vi "H5Sselect_hyperslab.vi"(4 "Count":u64[](array[numeric]), 5 "Block":u64[](array[numeric]), 6 "Start":u64[](array[numeric]), 7 "Stride":u64[](array[numeric]), 8 "error in (no error)":errorcluster, 10 "Operator":T1 items=["H5S_SELECT_NOOP"=-1, "H5S_SELECT_SET"=0, "H5S_SELECT_OR"=1, "H5S_SELECT_AND"=2, "H5S_SELECT_XOR"=3, "H5S_SELECT_NOTB"=4, "H5S_SELECT_NOTA"=5, "H5S_SELECT_APPEND"=6, "H5S_SELECT_PREPEND"=7], 11 "HDF5 Space Ref":T2) -> (0 "error out":errorcluster, 3 "HDF5 Ref out":T2)   [LabVIEW 2017]
doc: "Selects a hyperslab region to add to the current selected region."
uses:
  <vilib>/UPVI/lvhdf5/library.llb/HDF5 Ref.ctl
  <vilib>/UPVI/lvhdf5/dataspace.llb/H5S_seloper_t.ctl
  <vilib>/UPVI/lvhdf5/hdf5.dll
panel:
  # "LVHDF5 Toolkit\nCopyright (c) 2005-2013 by Jason D. Sommerville\nCopyright (c) 2014 by UPVI, LLC.\n\nThis use and distribution of this file is governed by the terms found in \nLICENSE.txt distributed with this toolkit and installed at\n <user.lib>\\_lvhdf5\\LICENSE.txt"
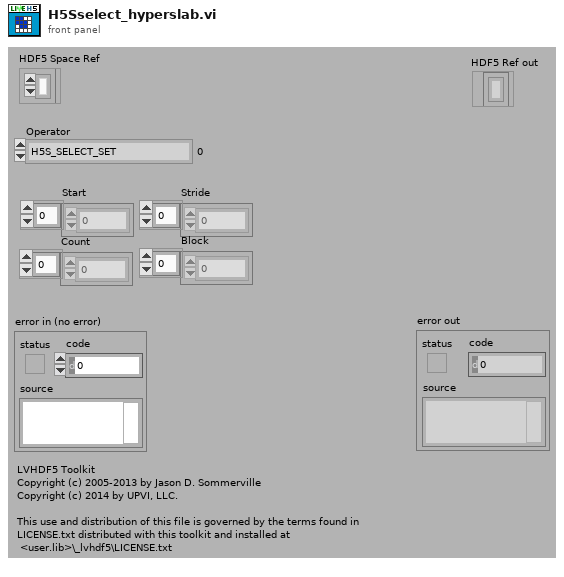
[diagram p1: front panel]
types:
  T1 = typedef "H5S_seloper_t.ctl" = i32
  T2 = typedef "HDF5 Ref.ctl" = refnum<k1>
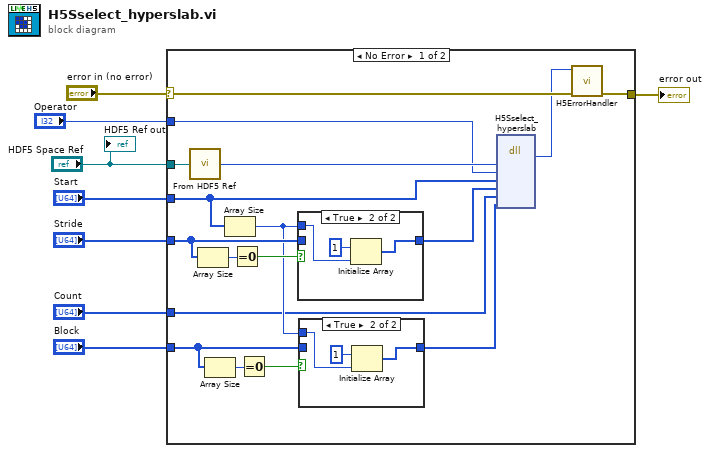
[diagram p0: block diagram]
diagram:
  n1 = case shown="No Error" "error in (no error)" {
    selector: "error in (no error)" -> [w25 w34]
    tunnel: [w24 w34] -> w7
    tunnel: "HDF5 Space Ref" -> [w23 _]
    tunnel: "Operator" -> [w20 _]
    tunnel: "Start" -> [w10 _]
    tunnel: "Stride" -> [w17 _]
    tunnel: "Count" -> [w12 _]
    tunnel: "Block" -> [w15 _]
    frame No Error {
      n2 = call <vilib>:"From HDF5 Ref.vi"("HDF5 Ref"=w23) -> ("I32"=w22:i32)
      n3 = Array Size(array=w17) -> (size(s)=w19:i32)
      n4 = Array Size(array=w15) -> (size(s)=w16:i32)
      n5 = Array Size(array=w10) -> (size(s)=w13:i32)
      n6 = Equal To 0?(x=w19) -> (x = 0?=w18:bool)
      n7 = Equal To 0?(x=w16) -> (x = 0?=w14:bool)
      n8 = case shown="True" w18 {
        tunnel: w13 -> [_ w33]
        tunnel: w17 -> [w30 _]
        tunnel: [w30 w31] -> w9
        frame False {
        }
        frame True {
          n9 = Initialize Array(u64 1 ("element"), w33) -> (w31:u64[])
        }
      }
      n10 = case shown="True" w14 {
        tunnel: w13 -> [_ w29]
        tunnel: w15 -> [w26 _]
        tunnel: [w26 w27] -> w11
        frame False {
        }
        frame True {
          n11 = Initialize Array(u64 1 ("element"), w29) -> (w27:u64[])
        }
      }
      n12 = dll-call lib="C:/Program Files/National Instruments/LabVIEW 2017/vi.lib/UPVI/lvhdf5/hdf5.dll" fn="H5Sselect_hyperslab"("space_id"=w22, "op"=w20, "start"=w10, "stride"=w9, "count"=w12, "block"=w11) -> ("return type"=w21:i32)  [unwired: 9 in, 2 out]
      n13 = call <vilib>:"H5ErrorHandler.vi"("error in (no error)"=w25, "herr_t"=w21) -> ("error out"=w24:errorcluster)  [unwired: 3 in, 4 out]
    }
    frame Error {
    }
  }
  "error out" <- w7
  "HDF5 Ref out" <- "HDF5 Space Ref"
